vi "replaceQueryTokens.vi"(8 "error in (no error)":errorcluster, 10 "Query In":string, 11 "Transaction in":refnum<class "Transaction.lvclass">) -> (0 "error out":errorcluster, 2 "Query Out":string, 3 "Transaction out":refnum<class "Transaction.lvclass">)   [LabVIEW 2020, in "Transaction.lvclass"]
uses:
  Transaction.lvclass
  Transaction.lvclass/Transaction.ctl
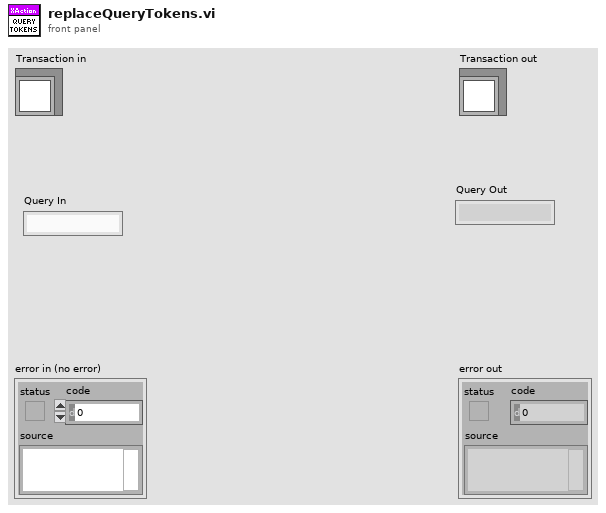
[diagram p1: front panel]
types:
  T1 = typedef "LVDateTimeRec.ctl" = cluster{"fractional second":dbl, "second":i32, "minute":i32, "hour":i32, "day of month":i32, "month":i32, "year":i32, "day of week":i32, "day of year":i32, "DST":i32}
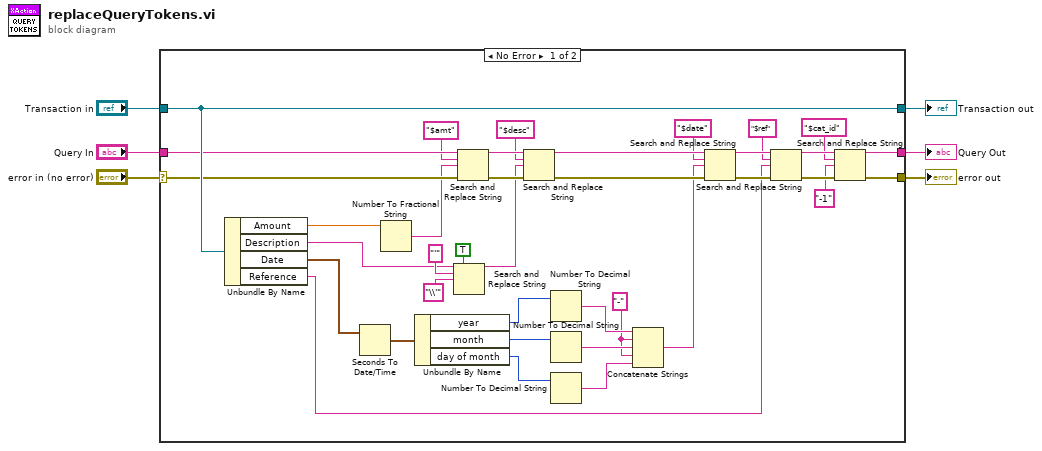
[diagram p0: block diagram]
diagram:
  n1 = case shown="No Error" "error in (no error)" {
    selector: "error in (no error)" -> [w42 w46]
    tunnel: [w40 w46] -> w5
    tunnel: [w43 w45] -> w3
    tunnel: "Transaction in" -> [w43 w45]
    tunnel: "Query In" -> [w41 w44]
    tunnel: [w31 w44] -> w1
    frame No Error {
      w18 = "-"
      n2 = Unbundle By Name(w43) -> ("Amount"=w24:dbl, "Description"=w23:string, "Date"=w12:timestamp, "Reference"=w10:string)
      n3 = Seconds To Date/Time(time stamp (now)=w12) -> (date time rec=w14:T1)  [unwired: 1 in]
      n4 = Number To Fractional String(number=w24) -> (F-format string=w30:string)  [unwired: 3 in]
      n5 = Unbundle By Name(w14) -> ("year"=w15:i32, "month"=w16:i32, "day of month"=w17:i32)
      n6 = Search and Replace String(replace all?=TRUE ("replace all? (F)"), input string=w23, search string="'", replace string="\\'") -> (result string=w22:string)  [unwired: 1 in, 6 out]
      n7 = Search and Replace String(input string=w41, search string="$amt", replace string=w30, error in=w42) -> (result string=w35:string, error out=w39:errorcluster)  [unwired: 4 in, 2 out]
      n8 = Search and Replace String(input string=w35, search string="$desc", replace string=w22, error in=w39) -> (result string=w34:string, error out=w38:errorcluster)  [unwired: 4 in, 2 out]
      n9 = Number To Decimal String(number=w15) -> (decimal integer string=w19:string)  [unwired: 1 in]
      n10 = Number To Decimal String(number=w16) -> (decimal integer string=w20:string)  [unwired: 1 in]
      n11 = Number To Decimal String(number=w17) -> (decimal integer string=w21:string)  [unwired: 1 in]
      n12 = Concatenate Strings(w19, w18, w20, w18, w21) -> (w11:string)
      n13 = Search and Replace String(input string=w34, search string="$date", replace string=w11, error in=w38) -> (result string=w33:string, error out=w37:errorcluster)  [unwired: 4 in, 2 out]
      n14 = Search and Replace String(input string=w33, search string="$ref", replace string=w10, error in=w37) -> (result string=w32:string, error out=w36:errorcluster)  [unwired: 4 in, 2 out]
      n15 = Search and Replace String(input string=w32, search string="$cat_id", replace string="-1" ("replace string (\"\")"), error in=w36) -> (result string=w31:string, error out=w40:errorcluster)  [unwired: 4 in, 2 out]
    }
    frame Error {
    }
  }
  "error out" <- w5
  "Transaction out" <- w3
  "Query Out" <- w1
